vi "Enqueue File.vi"(10 "filepath":path, 11 "Blocks queue":refnum<queue>) -> (2 "error out":errorcluster)   [LabVIEW 2013, in "MD5.lvlib" / "MD5.lvclass"]
uses:
  MD5.lvclass
  Data-vector.ctl
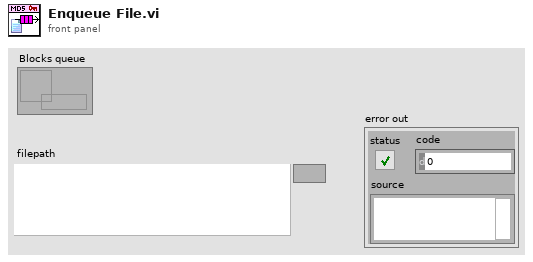
[diagram p1: front panel]
types:
  T1 = enum16{"open", "replace", "create", "open or create", "replace or create", "replace or create with confirmation"}
  T2 = typedef "MD5.lvlib/MD5.lvclass/Data-vector.ctl" = cluster{"Data[ ]":u8[], "end":bool}
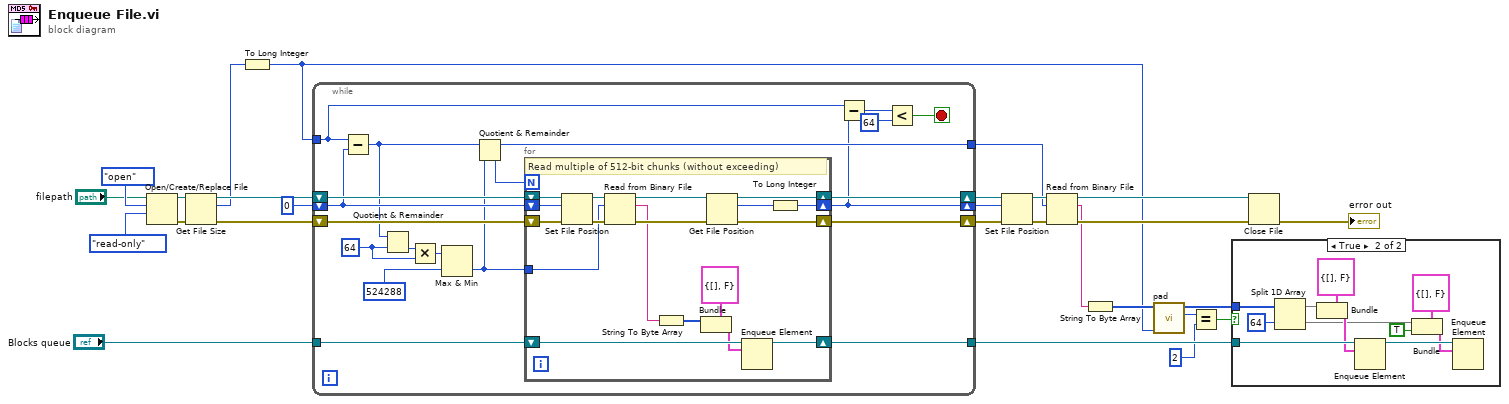
[diagram p0: block diagram]
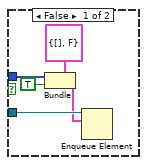
[diagram p2: hidden frame]
diagram:
  n1 = Open/Create/Replace File(file path (use dialog)="filepath", operation (0:open)=T1."open", access (0:read/write)=enum16{"read/write", "read-only", "write-only"}."read-only") -> (refnum out=w17:refnum<file>, error out=w18:errorcluster)  [unwired: 3 in, 1 out]
  n2 = Get File Size(file=w17, error in=w18) -> (refnum out=w16:refnum<file>, size (in bytes)=w2:i64, 0:w14:errorcluster)
  n3 = To Long Integer(number=w2) -> (32bit integer=w1:i32)
  n4 = while {
    tunnel: "Blocks queue" -> [w47]
    tunnel: [w46] -> w23
    shift-right: [w31] -> w12
    shift-left: 0 ("offset") -> [w41]
    shift-right: [w43] -> w13
    shift-left: w16 -> [w45]
    shift-right: [w42] -> w11
    shift-left: w14 -> [w44]
    tunnel: w1 -> [w32]
    tunnel: [w33] -> w3
    stop <- w28 stop-if-true
    w34 = 64 ("y")
    n5 = Subtract(x=w32, y=w41) -> (x-y=w40:i32)
    n6 = Quotient & Remainder(x=w40, y=w34) -> (floor(x/y)=w39:i32)  [unwired: 1 out]
    n7 = Multiply(x=w39, y=w34) -> (x*y=w38:i32)
    n8 = Max & Min(x=w38, y=524288) -> (min(x,y)=w35:i32)  [unwired: 1 out]
    n9 = Quotient & Remainder(x=w40, y=w35) -> (x-y*floor(x/y)=w33:i32, floor(x/y)=w36:i32)
    n10 = for {
      N: w36 -> [_]
      shift-right: [w56] -> w43
      shift-left: w45 -> [w59]
      shift-right: [w64] -> w46
      shift-left: w47 -> [w65]
      shift-right: [w53] -> w31
      shift-left: w41 -> [w58]
      tunnel: w35 -> [w51]
      shift-right: [w54] -> w42
      shift-left: w44 -> [w55]
      # "Read multiple of 512-bit chunks (without exceeding)"
      n11 = Set File Position(offset (in bytes) (0)=w58, refnum=w59, error in=w55) -> (refnum out=w60:refnum<file>, error out=w61:errorcluster)  [unwired: 1 in]
      n12 = Read from Binary File(8:w61, 10:w51, 11:w60) -> (0:w63:errorcluster, 2:w52:string, 3:w62:refnum<file>)  [unwired: 3 in, 1 out]
      n13 = String To Byte Array(string=w52) -> (unsigned byte array=w48:u8[])
      n14 = Bundle(cluster=T2 {"Data[ ]"=[], "end"=FALSE}, "Data[ ]"=w48) -> (w49:T2)  [unwired: 1 in]
      n15 = Get File Position(4:w63, 7:w62) -> (0:w54:errorcluster, 2:w57:i64, 3:w56:refnum<file>)
      n16 = Enqueue Element(queue=w65, element=w49) -> (queue out=w64:refnum<queue>)  [unwired: 2 in, 2 out]
      n17 = To Long Integer(number=w57) -> (32bit integer=w53:i32)
    }
    n18 = Subtract(x=w32, y=w31) -> (x-y=w30:i32)
    n19 = Less?(x=w30, y=64) -> (x < y?=w28:bool)
  }
  n20 = Set File Position(offset (in bytes) (0)=w12, refnum=w13, error in=w11) -> (refnum out=w10:refnum<file>, error out=w9:errorcluster)  [unwired: 1 in]
  n21 = Read from Binary File(8:w9, 10:w3, 11:w10) -> (0:w7:errorcluster, 2:w6:string, 3:w8:refnum<file>)  [unwired: 3 in, 1 out]
  n22 = String To Byte Array(string=w6) -> (unsigned byte array=w5:u8[])
  n23 = call "pad.vi"("data length"=w1, "Last Block"=w5) -> ("blocks"=w25:i32, "Padding"=w24:u8[])  [unwired: 8 in]
  n24 = Equal?(x=w25, y=2) -> (x = y?=w26:bool)
  n25 = case shown="True" w26 {
    tunnel: w23 -> [w67 w81]
    tunnel: w24 -> [w69 w80]
    frame False {
      n26 = Bundle(cluster=T2 {"Data[ ]"=[], "end"=FALSE}, "Data[ ]"=w69, "end"=TRUE) -> (w66:T2)
      n27 = Enqueue Element(queue=w67, element=w66) -> ()  [unwired: 2 in, 3 out]
    }
    frame True {
      n28 = Split 1D Array(array=w80, index=64) -> (first subarray=w76:u8[], second subarray=w73:u8[])
      n29 = Bundle(cluster=T2 {"Data[ ]"=[], "end"=FALSE}, "Data[ ]"=w76) -> (w78:T2)  [unwired: 1 in]
      n30 = Enqueue Element(queue=w81, element=w78) -> (queue out=w75:refnum<queue>)  [unwired: 2 in, 2 out]
      n31 = Bundle(cluster=T2 {"Data[ ]"=[], "end"=FALSE}, "Data[ ]"=w73, "end"=TRUE) -> (w71:T2)
      n32 = Enqueue Element(queue=w75, element=w71) -> ()  [unwired: 2 in, 3 out]
    }
  }
  n33 = Close File(refnum=w8, error in=w7) -> (error out=→"error out":errorcluster)  [unwired: 1 out]
